vi "Reset_coutout.vi"(8 "error in (no error)":errorcluster caption="错误输入（无错误）", 10 "测试信息 2":refnum<vi>, 11 "configuration file path":path caption="配置文件的路径") -> (0 "error out":errorcluster caption="错误输出", 3 "添加的路径":path)   [LabVIEW 2018]
uses:
  <vilib>/Utility/config.llb/Write Key (String).vi
  <vilib>/Utility/config.llb/NI_LVConfig.lvlib
panel:
  in  "测试信息":i32(listbox)
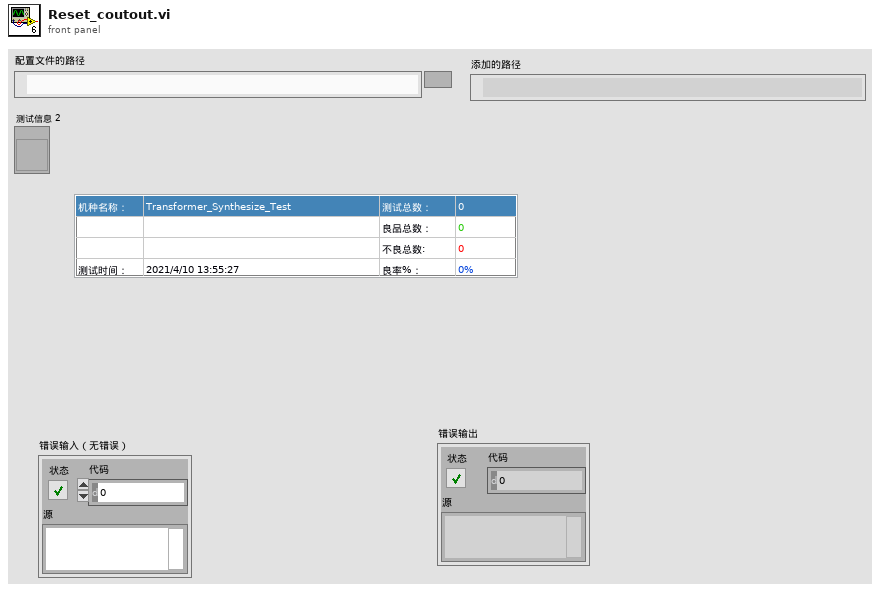
[diagram p1: front panel]
types:
  T1 = typedef "NI_LVConfig.lvlib/Config Data RefNum.ctl" = refnum<k1>
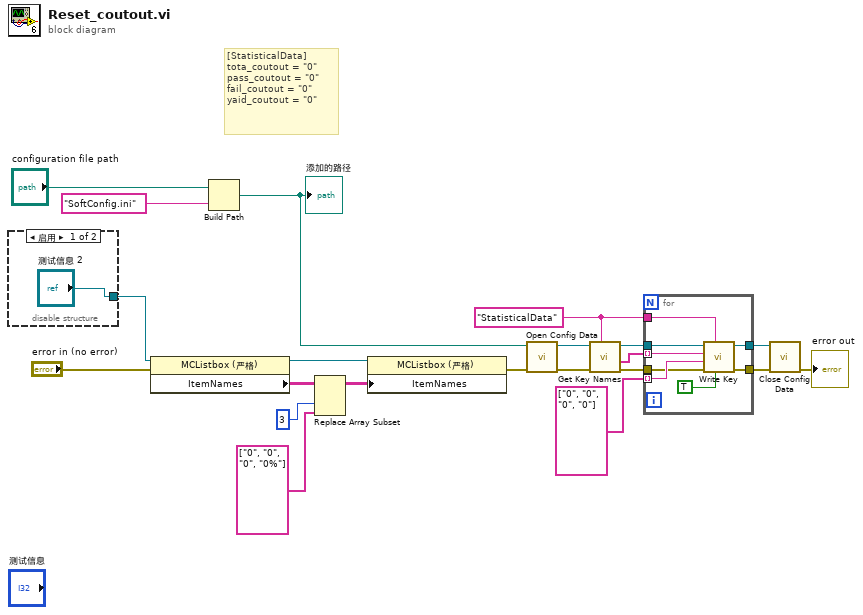
[diagram p0: block diagram]
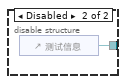
[diagram p2: hidden frame]
diagram:
  w12 = "StatisticalData" ("section")
  # "[StatisticalData]\ntota_coutout = \"0\"\npass_coutout = \"0\"\nfail_coutout = \"0\"\nyaid_coutout = \"0\""
  n1 = disable-structure shown="启用" {
    disable-tunnel: ["测试信息 2" w23] -> w15
    frame Enabled {
    }
    frame Disabled {
      n2 = control-ref of="测试信息"() -> (w23:refnum<vi>)
    }
  }
  n3 = property class="MCListbox (严格)"(reference=w15, error in="error in (no error)") -> (reference out=w1:refnum<vi>, "ItemNames"=w5:string[][])  [unwired: 1 out]
  n4 = Build Path(base path="configuration file path", name or relative path="SoftConfig.ini" ("名称或相对路径")) -> (appended path=w8:path)
  "添加的路径" <- w8
  n5 = Replace Array Subset(array=w5, new element=string[] ["0", "0", "0", "0%"] ("ItemNames"), index (col)=3 ("禁用的索引 (列)")) -> (w4:string[][])  [unwired: 1 in]
  n6 = property class="MCListbox (严格)"(reference=w1, "ItemNames"=w4) -> (error out=w6:errorcluster)  [unwired: 1 in, 1 out]
  n7 = call <vilib>:"Open Config Data.vi"("error in (no error)"=w6, "configuration file path"=w8) -> ("error out"=w16:errorcluster, "refnum"=w14:T1)  [unwired: 7 in, 1 out]
  n8 = call <vilib>:"Get Key Names.vi"("section"=w12, "error in (no error)"=w16, "refnum"=w14) -> ("error out"=w17:errorcluster, "key names"=w13:string[], "refnum out"=w11:T1)  [unwired: 5 in, 1 out]
  n9 = for {
    tunnel: w13 -> [w30] mode=indexing
    tunnel: w12 -> [w31]
    tunnel: w11 -> [w29]
    tunnel: string[] ["0", "0", "0", "0"] ("ItemNames") -> [w28] mode=indexing
    tunnel: w17 -> [w27]
    tunnel: [w26] -> w20
    tunnel: [w24] -> w19
    n10 = call-poly <vilib>:"Write Key.vi"("write raw string? (F)"=TRUE, "section"=w31, "error in (no error)"=w27, "value"=w28, "key"=w30, "refnum"=w29) -> ("error out"=w26:errorcluster, "refnum out"=w24:T1)  [unwired: 3 in, 1 out]
  }
  n11 = call <vilib>:"Close Config Data.vi"("error in (no error)"=w20, "refnum"=w19) -> ("error out"=→"error out":errorcluster)  [unwired: 8 in, 1 out]
